vi "2023 Arm Case Stmt.vi"(2 "error in (no error)":errorcluster, 3 "Boolean":bool, 4 "joystickInput":dbl) -> (0 "error out":errorcluster, 1 "Sensor Position":dbl)   [LabVIEW 2020]
uses:
  <vilib>/Rock Robotics/Network Tables/NT Read Number.vi
  <vilib>/Rock Robotics/WPI/ThirdParty/REV Robotics/REVLib/Typedef/Spark MAX Control Type.ctl
  <vilib>/Rock Robotics/Network Tables/NT Write Number.vi
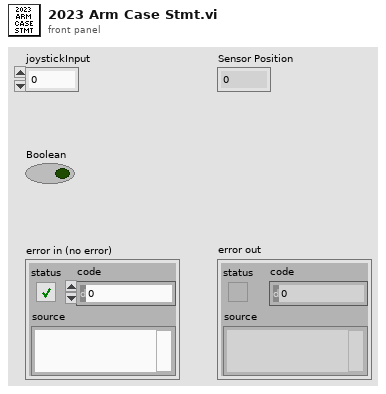
[diagram p1: front panel]
types:
  T1 = typedef "WPI_MotorControlDeviceRef.ctl" = cluster{"DeviceStatus":errorcluster, "Type":T2, "PWM":cluster{"PWM Channel":T3, "DeadBand":T4}, "CAN":cluster{"Device Number":u8, "SetOutput VI Ref":variant, "GetOutput VI Ref":variant, "Enable VI Ref":variant, "Disable VI Ref":variant, "Data":variant}, "Invert":bool, "DIO PWM":cluster{"PWM \"Enable\" Channel":T3, "DIOChannel":T5, "PWM Rate":dbl}}
  T2 = typedef "WPI_MotorControlType.ctl" = enum16{"PWM", "CAN", "DIO PWM"}
  T3 = typedef "FPGA_DIOPWMChannel.ctl" = enum8{"PWM 0", "PWM 1", "PWM 2", "PWM 3", "PWM 4", "PWM 5", "PWM 6", "PWM 7", "PWM 8", "PWM 9", "PWM MXP 0", "PWM MXP 1", "PWM MXP 2", "PWM MXP 3", "PWM MXP 4", "PWM MXP 5", "PWM MXP 6", "PWM MXP 7", "PWM MXP 8", "PWM MXP 9", "Invalid"}
  T4 = typedef "WPI_PWMDeadband.ctl" = cluster{"Name":string, "maxPositivePwm":i32, "minPositivePwm":i32, "centerPwm":i32, "maxNegativePwm":i32, "minNegativePwm":i32, "angularRange":u16}
  T5 = typedef "FPGA_DIOChannel.ctl" = enum8{"DIO 0", "DIO 1", "DIO 2", "DIO 3", "DIO 4", "DIO 5", "DIO 6", "DIO 7", "DIO 8", "DIO 9", "DIO MXP 0", "DIO MXP 1", "DIO MXP 2", "DIO MXP 3", "DIO MXP 4", "DIO MXP 5", "DIO MXP 6", "DIO MXP 7", "DIO MXP 8", "DIO MXP 9", "DIO MXP 10", "DIO MXP 11", "DIO MXP 12", "DIO MXP 13", "DIO MXP 14", "DIO MXP 15", "SPI Port CS1", "SPI Port CS2", "SPI Port CS3", "SPI Port MISO", "SPI Port MOSI", "Invalid"}
  T6 = typedef "Spark MAX Control Type.ctl" = enum16{"Percent VBus", "Voltage", "Velocity", "Position", "Smart Motion", "Current", "Smart Velocity"}
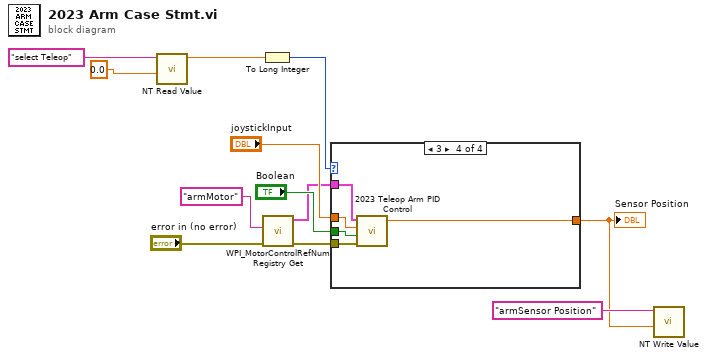
[diagram p0: block diagram]
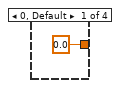
[diagram p2: hidden frame]
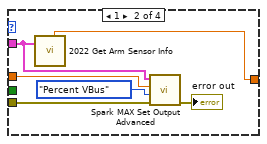
[diagram p3: hidden frame]
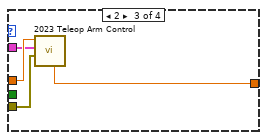
[diagram p4: hidden frame]
diagram:
  n1 = call-poly <vilib>:"NT Read Value.vi"("default value"=0.0, "name"="select Teleop") -> ("value"=w9:dbl)  [unwired: 7 in, 2 out]
  n2 = To Long Integer(number=w9) -> (32bit integer=w10:i32)
  n3 = call <vilib>:"WPI_MotorControlRefNum Registry Get.vi"("error in (no error)"="error in (no error)", "refnum name"="armMotor") -> ("error out"=w2:errorcluster, "MotorControlDevRef"=w3:T1)  [unwired: 8 in]
  n4 = case shown="3" w10 {
    tunnel: [0.0 ("Sensor Position") w14 w23 w27] -> w5
    tunnel: "joystickInput" -> [_ w18 w22 w28]
    tunnel: "Boolean" -> [_ _ _ w26]
    tunnel: w3 -> [_ w15 w21 w25]
    tunnel: w2 -> [_ w16 w20 w24]
    frame 0, Default {
    }
    frame 1 {
      n5 = call "2022 Get Arm Sensor Info.vi"("MotorControlDevRef"=w15) -> ("Sensor Position"=w14:dbl)  [unwired: 1 in, 4 out]
      n6 = call <vilib>:"Spark MAX Set Output Advanced.vi"("error in (no error)"=w16, "Control Mode"=Spark_MAX_Control_Type."Percent VBus", "Setpoint"=w18, "MotorControlDevRef"=w15) -> ("error out"=→"error out":errorcluster)  [unwired: 6 in, 1 out]
    }
    frame 2 {
      n7 = call "2023 Teleop Arm Control.vi"("error in (no error)"=w20, "MotorControlDevRef"=w21, "Joystick Y Axis"=w22) -> ("Sensor Position"=w23:dbl)  [unwired: 7 in, 1 out]
    }
    frame 3 {
      n8 = call "2023 Teleop Arm PID Control.vi"("error in (no error)"=w24, "reinitialize? (F)"=w26, "Joystick Y Axis"=w28, "MotorControlDevRef"=w25) -> ("Sensor Position"=w27:dbl)  [unwired: 2 out]
    }
  }
  "Sensor Position" <- w5
  n9 = call-poly <vilib>:"NT Write Value.vi"("value"=w5, "name"="armSensor Position") -> ()  [unwired: 9 in, 1 out]
